vi "ImageToDvrU32_2D.vi"(7 "Optional Rectangle":T4, 8 "error in":errorcluster, 9 "Step Sizes":T1={"X Step Size"=1, "Y Step Size"=1}, 10 "Include Border":bool, 11 "Image Reference In":T3) -> (0 "error out":errorcluster, 1 "Line Info":T2, 2 "EDVR 2D U32":refnum<data-value>, 3 "Image Reference Out":T3)   [LabVIEW 2020, in "OpenLvVision_Image.lvlib" / "DataAccess.lvlib"]
doc: "Returns a DVR (Data Value Reference) to the image data, allowing direct manipulation without copying. \nDelete the DVR after use."
uses:
  DataAccess.lvlib
  TypeDef/RectangleI32.ctl
  Management/TypeDef/Image.ctl
  TypeDef/LineInfo.ctl
  TypeDef/StepSizes.ctl
  <vilib>/vision/EDVR.llb/IMAQ ImageToEDVR 2D U32.vi
  Management/Management.lvlib
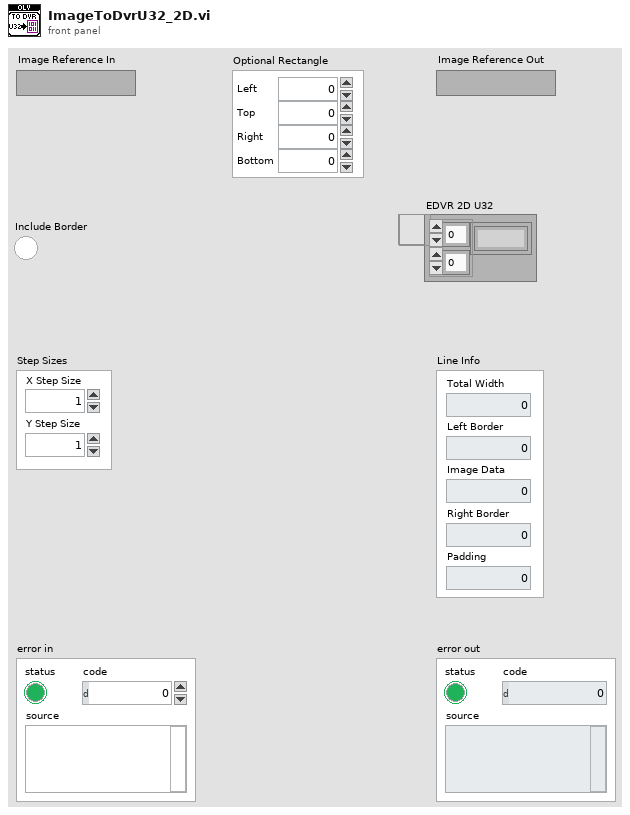
[diagram p1: front panel]
types:
  T1 = typedef "OpenLvVision_Image.lvlib/DataAccess.lvlib/StepSizes.ctl" = cluster{"X Step Size":u32, "Y Step Size":u32}
  T2 = typedef "OpenLvVision_Image.lvlib/DataAccess.lvlib/LineInfo.ctl" = cluster{"Total Width":u32, "Left Border":u32, "Image Data":u32, "Right Border":u32, "Padding":u32}
  T3 = typedef "OpenLvVision_Image.lvlib/Management.lvlib/Image.ctl" = refnum<image>
  T4 = typedef "OpenLvVision_Image.lvlib/DataAccess.lvlib/RectangleI32.ctl" = cluster{"Left":i32, "Top":i32, "Right":i32, "Bottom":i32}
  T5 = cluster{"Total Width":u32, "Left Border":u32, "Image Data":u32, "Right Border":u32, "Padding":u32}
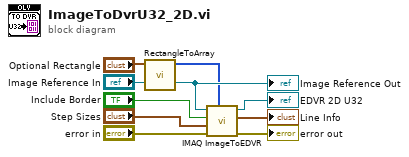
[diagram p0: block diagram]
diagram:
  n1 = call "RectangleToArray.vi"("Optional Rectangle"="Optional Rectangle") -> ("Array"=w5:i32[])  [unwired: 10 in]
  n2 = call-poly <vilib>:"IMAQ ImageToEDVR.vi"("Optional Rectangle"=w5, "error out"="error in", "Step Sizes"="Step Sizes", "Include Border Pixels (F)"="Include Border", "Image"="Image Reference In") -> ("error out"=→"error out":errorcluster, "Line Info"=→"Line Info":T5, "EDVR 2D U32"=→"EDVR 2D U32":refnum<data-value>)  [unwired: 4 in]
  "Image Reference Out" <- "Image Reference In"
